vi "LVClasse_HasoConfig dtor.vi"(0 "HasoConfig in":refnum<class "HasoConfig.lvclass">, 11 "error in (no error)":errorcluster) -> (4 "HasoConfig out":refnum<class "HasoConfig.lvclass">, 15 "error out":errorcluster)   [LabVIEW 2020, in "HasoConfig.lvclass"]
doc: "Surface destructor.\n\n--------------------------------------------------------------------------------\n\n<B>surfaceIn </B> : Surface object.\n<B>surfaceOut </B> : Surface object.\n<B>ErrorIn </B> : Error\n<B>ErrorOut </B> : Error\n\n--------------------------------------------------------------------------------"
uses:
  HasoConfig.lvclass
  HasoConfig.lvclass/HasoConfig.ctl
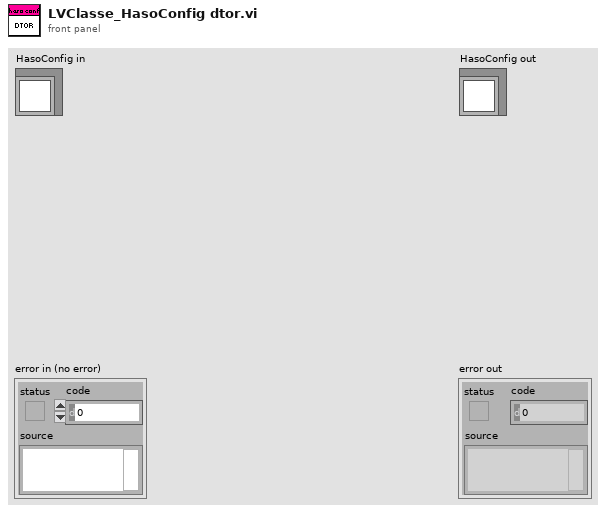
[diagram p1: front panel]
types:
  T1 = typedef "Handle creation.ctl" = enum16{"By ctor", "By write function"}
  T2 = typedef "ClassID.ctl" = i64
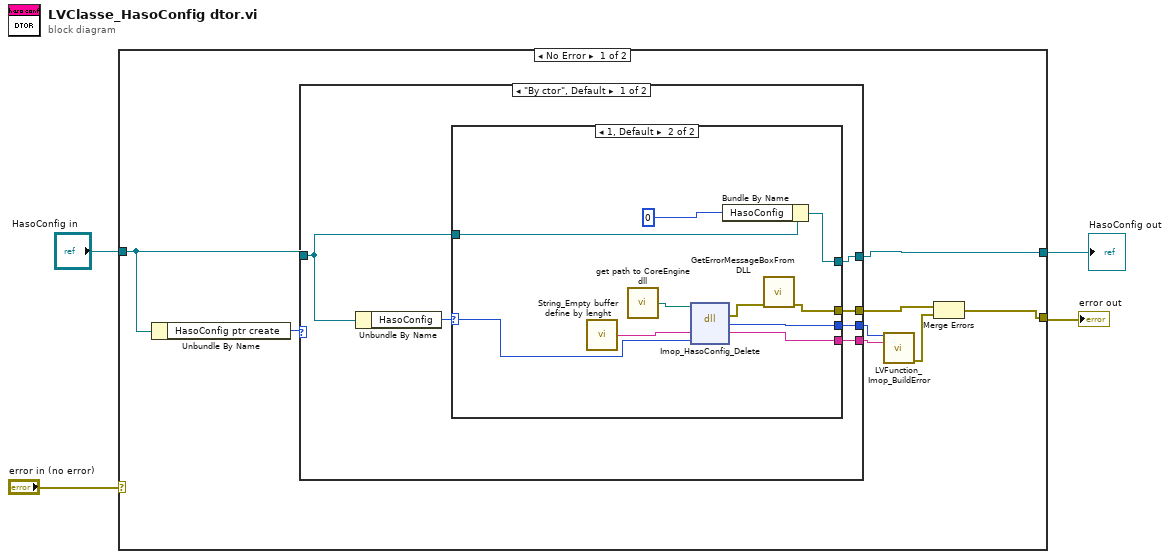
[diagram p0: block diagram]
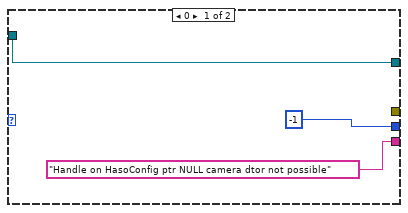
[diagram p2: hidden frame]
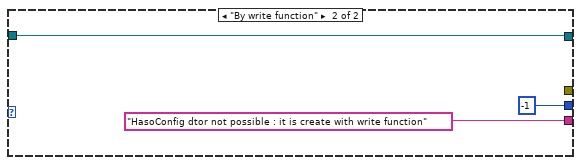
[diagram p3: hidden frame]
diagram:
  n1 = case shown="No Error" "error in (no error)" {
    selector: "error in (no error)" -> [_ w35]
    tunnel: "HasoConfig in" -> [w10 w36]
    tunnel: [w5 w36] -> w2
    tunnel: [w6 w35] -> w1
    frame No Error {
      n2 = Unbundle By Name(w10) -> ("HasoConfig ptr create"=w9:T1)
      n3 = case shown="\"By ctor\", Default" w9 {
        tunnel: [w18 "HasoConfig dtor not possible : it is create with write function" ("message")] -> w12
        tunnel: [w17 -1] -> w11
        tunnel: w10 -> [w15 w32]
        tunnel: [w16 w32] -> w5
        tunnel: [w13 _] -> w8
        frame "By ctor", Default {
          n4 = Unbundle By Name(w15) -> ("HasoConfig"=w14:T2)
          n5 = case shown="1, Default" w14 {
            selector: w14 -> [_ w28]
            tunnel: ["Handle on HasoConfig ptr NULL camera dtor not possible" ("message") w30] -> w18
            tunnel: [-1 w29] -> w17
            tunnel: w15 -> [w19 w24]
            tunnel: [w19 w23] -> w16
            tunnel: [_ w22] -> w13
            frame 0 {
            }
            frame 1, Default {
              n6 = call "String_Empty buffer define by lenght.vi"() -> ("Empty buffer"=w31:string)  [unwired: 1 in]
              n7 = call "get path to CoreEngine dll.vi"() -> ("path to wavekit library"=w27:path)  [unwired: 14 in, 1 out]
              n8 = dll-call lib="D:/soft/HASO_v3/SVN_trunk/ImOpCoreEngine4_LV2011/DLLs/c_interface_vc100.dll" fn="Imop_HasoConfig_Delete"(path in=w27, "message"=w31, "HasoConfig"=w28) -> (error out=w26:errorcluster, "return type"=w29:i32, "message"=w30:string)  [unwired: 3 in, 1 out]
              n9 = Bundle By Name(cluster=w24, "HasoConfig"=u32 0 ("HasoEgine")) -> (w23:refnum<class "HasoConfig.lvclass">)
              n10 = call "GetErrorMessageBoxFromDLL.vi"("error IN"=w26) -> ("error OUT"=w22:errorcluster)  [unwired: 10 in]
            }
          }
        }
        frame "By write function" {
        }
      }
      n11 = call "LVFunction_Imop_BuildError.vi"("code"=w11, "String to Prepend to source (\"\")"=w12) -> ("error out"=w7:errorcluster)  [unwired: 13 in]
      n12 = Merge Errors(w8, w7) -> (w6:errorcluster)
    }
    frame Error {
    }
  }
  "error out" <- w1
  "HasoConfig out" <- w2
